vi "Actor Setup.vi"(10 "Actor":refnum<class "Actor.lvclass">, 11 "Dev Actor in":refnum<class "Dev Actor.lvclass">) -> (3 "Dev Actor out":refnum<class "Dev Actor.lvclass">)   [LabVIEW 2021, in "Dev Actor.lvlib" / "Dev Actor.lvclass"]
uses:
  Dev Actor.lvclass
  <vilib>/jettl/jettl/jettl/Actor/Actor.lvclass
  Dev Actor.lvclass/Dev Actor.ctl
  <vilib>/jettl/jettl/Msgs/Actor Destroy/Actor Destroy Msg Strategy/Actor Destroy Msg Strategy.lvclass
  C:/Program Files/National Instruments/LabVIEW 2021/vi.lib/jettl/jettl/jettl/Msg Strategy/Msg Strategy.lvclass
  Panel/Panel.lvclass
  Dev Actor Panel/Dev Actor Panel.lvclass
  C:/git/jettl/examples/Dev Actor/Panel/Panel.lvclass
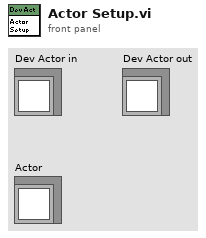
[diagram p1: front panel]
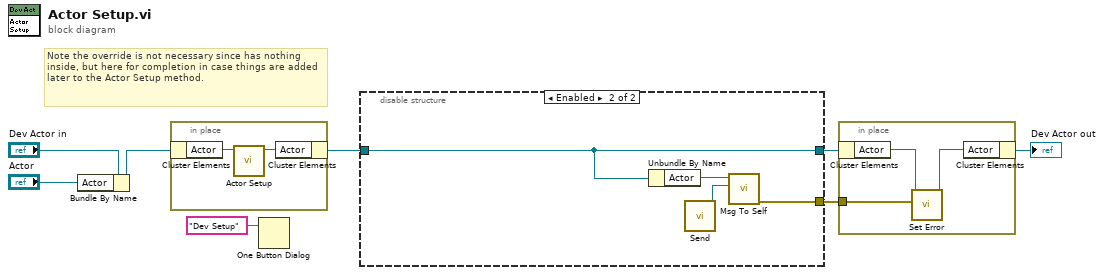
[diagram p0: block diagram]
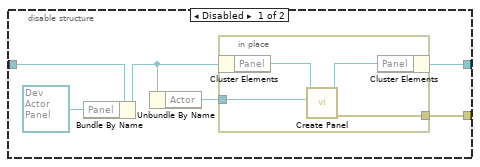
[diagram p2: hidden frame]
diagram:
  # "Note the override is not necessary since has nothing inside, but here for completion in case things are added later to the Actor Setup method."
  n1 = Bundle By Name(cluster="Dev Actor in", "Actor"="Actor") -> (w5:refnum<class "Dev Actor.lvclass">)
  n2 = in-place {
    n3 = in-place-cluster #1(w5) -> ("Actor"=w9:refnum<class "Actor.lvclass">)
    n4 = call-dynamic "Actor Setup.vi"("Actor in"=w9) -> ("Actor out"=w10:refnum<class "Actor.lvclass">)  [unwired: 10 in]
    n5 = in-place-cluster #1("Actor"=w10) -> (w4:refnum<class "Dev Actor.lvclass">)
  }
  n6 = One Button Dialog(message="Dev Setup") -> ()  [unwired: 1 in, 1 out]
  n7 = disable-structure shown="Enabled" {
    disable-tunnel: w4 -> [w13 w24]
    disable-tunnel: [w12 w24] -> w3
    disable-tunnel: [w11 w21] -> w1
    frame Disabled {
      n8 = Bundle By Name(cluster=w13, "Panel"=refnum<class "Dev Actor Panel.lvclass"> refnum ("ABD Panel.lvclass")) -> (w15:refnum<class "Dev Actor.lvclass">)
      n9 = Unbundle By Name(w15) -> ("Actor"=w16:refnum<class "Actor.lvclass">)
      n10 = in-place {
        in-place-border: [w18] -> w11
        in-place-border: w16 -> [w17]
        n11 = in-place-cluster #2(w15) -> ("Panel"=w20:refnum<class "Panel.lvclass">)
        n12 = call "Create Panel.vi"("Actor"=w17, "Panel in"=w20) -> ("error out"=w18:errorcluster, "Panel out"=w19:refnum<class "Panel.lvclass">)  [unwired: 8 in]
        n13 = in-place-cluster #2("Panel"=w19) -> (w12:refnum<class "Dev Actor.lvclass">)
      }
    }
    frame Enabled {
      n14 = Unbundle By Name(w24) -> ("Actor"=w23:refnum<class "Actor.lvclass">)
      n15 = call <vilib>:"Send.vi"() -> ("Actor Destroy Msg Strategy out"=w22:refnum<class "Actor Destroy Msg Strategy.lvclass">)  [unwired: 11 in]
      n16 = call-dynamic "Msg To Self.vi"("Msg"=w22, "Actor in"=w23) -> ("error out"=w21:errorcluster)  [unwired: 9 in]
    }
  }
  n17 = in-place {
    in-place-border: w1 -> [w25]
    n18 = in-place-cluster #3(w3) -> ("Actor"=w27:refnum<class "Actor.lvclass">)
    n19 = call-dynamic "Set Error.vi"("Error"=w25, "Actor in"=w27) -> ("Actor out"=w26:refnum<class "Actor.lvclass">)  [unwired: 9 in]
    n20 = in-place-cluster #3("Actor"=w26) -> (→"Dev Actor out":refnum<class "Dev Actor.lvclass">)
  }
